vi "SputterTcpSample.vi"() -> ()   [LabVIEW 2021]
doc: "スパッタ制御PC用TCP通信サンプル"
uses:
  SubVI/HallMeasurementStatus.ctl
  SubVI/TcpCommunicationClientCMD.ctl
panel:
  in  "S2_Start":bool
  in  "S2_DataFilePath":path=path "S2_DataFile"
  out "S2_SettingFilePath":path
  out "S2_SampleName":string
  in  "S2_Status":T1
  out "TcpOK?":bool
  in  "S1_Start":bool
  in  "S1_DataFilePath":path=path "S1_DataFile"
  out "S1_SettingFilePath":path
  out "S1_SampleName":string
  in  "S1_Status":T1
  out "ReadData":string
  in  "Send Data":string
  in  "Send":bool
  in  "ポート":u16=8501
  in  "中央PCアドレス":string="localhost"
  in  "停止":bool
  # "スパッタ制御PC用TCP通信サンプル"
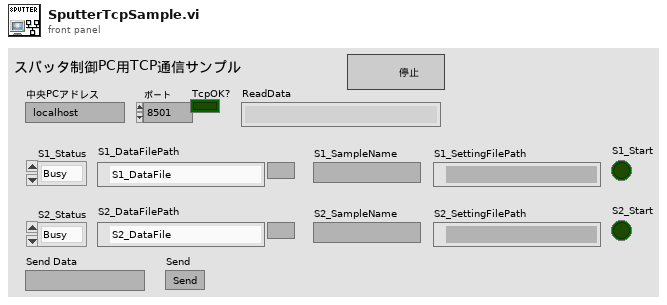
[diagram p1: front panel]
types:
  T1 = typedef "HallMeasurementStatus.ctl" = enum16{"Busy", "Ready", "Done", "Error"}
  T2 = typedef "TcpCommunicationClientCMD.ctl" = enum16{"Read", "Write", "Close"}
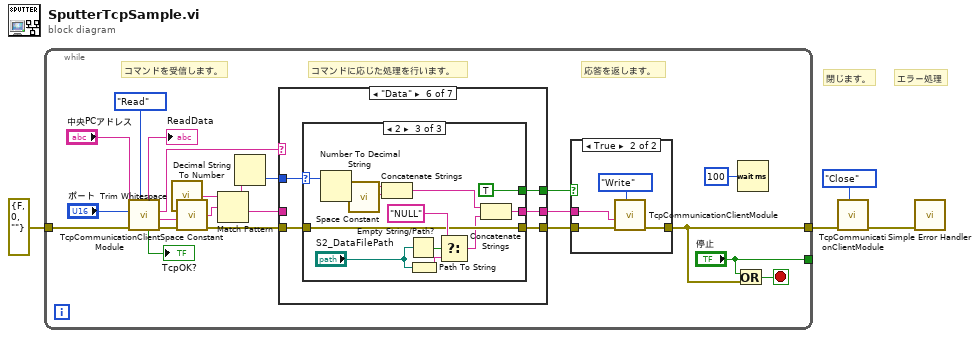
[diagram p0: block diagram]
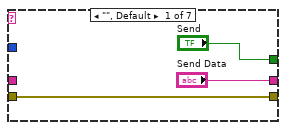
[diagram p3: hidden frame]
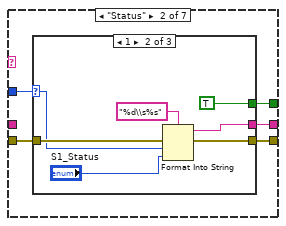
[diagram p4: hidden frame]
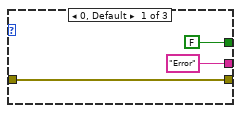
[diagram p5: hidden frame]
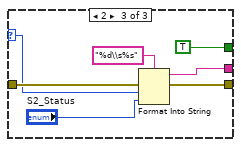
[diagram p6: hidden frame]
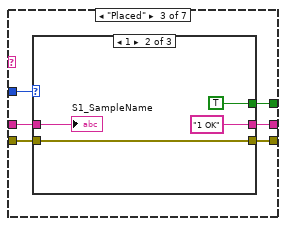
[diagram p7: hidden frame]
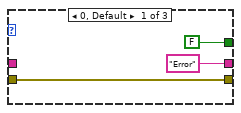
[diagram p8: hidden frame]
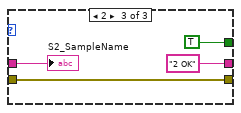
[diagram p9: hidden frame]
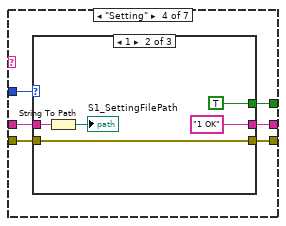
[diagram p10: hidden frame]
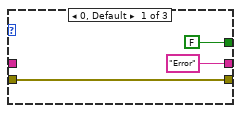
[diagram p11: hidden frame]
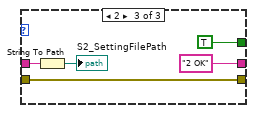
[diagram p12: hidden frame]
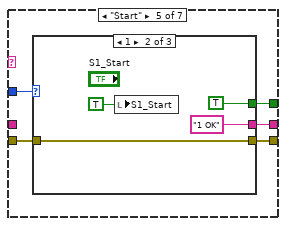
[diagram p13: hidden frame]
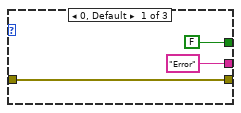
[diagram p14: hidden frame]
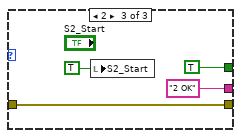
[diagram p15: hidden frame]
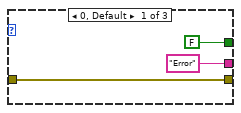
[diagram p16: hidden frame]
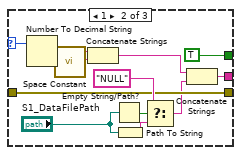
[diagram p17: hidden frame]
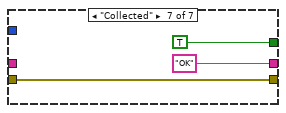
[diagram p18: hidden frame]
diagram:
  # "エラー処理"
  # "閉じます。"
  n1 = while {
    tunnel: ["停止"] -> _
    tunnel: [w14] -> w2
    tunnel: errorcluster {"status"=FALSE, "code"=0, "source"=""} ("エラー入力（エラーなし）") -> [w21]
    stop <- w25 stop-if-true
    # "応答を返します。"
    # "コマンドに応じた処理を行います。"
    # "コマンドを受信します。"
    n2 = call "TcpCommunicationClientModule.vi"("TcpCommunicationClientCMD"=TcpCommunicationClientCMD."Read", "エラー入力（エラーなし）"=w21, "ポート"="ポート", "アドレス"="中央PCアドレス") -> ("エラー出力"=w23:errorcluster, "Data"=w7:string, "Command"=w12:string, "TcpOK?"=→"TcpOK?":bool, "ReadData"=→"ReadData":string)  [unwired: 3 in]
    n3 = call <vilib>:"Trim Whitespace.vi"("string"=w7) -> ("trimmed string"=w8:string)  [unwired: 1 in]
    n4 = call <vilib>:"Space Constant.vi"() -> ("String"=w9:string)
    n5 = Match Pattern(string=w8, regular expression=w9) -> (before substring=w10:string, after substring=w6:string)  [unwired: 1 in, 2 out]
    n6 = Decimal String To Number(string=w10) -> (number=w5:i32)  [unwired: 2 in, 1 out]
    n7 = case shown="\"Data\"" w12 {
      tunnel: w6 -> [_ _ w59 w76 _ _ _]
      tunnel: ["Send Data" w38 w60 w77 w95 w111 "OK" ("Send Data")] -> w16
      tunnel: ["Send" w35 w61 w78 w96 w112 TRUE ("Send")] -> w17
      tunnel: w23 -> [w31 w37 w56 w73 w92 w109 w141]
      tunnel: [w31 w36 w57 w74 w93 w110 w141] -> w15
      tunnel: w5 -> [_ w34 w58 w75 w94 w108 _]
      frame "", Default {
      }
      frame "Status" {
        n8 = case shown="1" w34 {
          selector: w34 -> [_ w42 w50]
          tunnel: ["Error" w47 w55] -> w38
          tunnel: w37 -> [w41 w45 w53]
          tunnel: [w41 w44 w52] -> w36
          tunnel: [FALSE ("Send") TRUE ("Send") TRUE ("Send")] -> w35
          frame 0, Default {
          }
          frame 1 {
            n9 = Format Into String(format string="%d\\s%s" ("形式文字列"), error in=w45, w42, "S1_Status") -> (resulting string=w47:string, error out=w44:errorcluster)  [unwired: 1 in]
          }
          frame 2 {
            n10 = Format Into String(format string="%d\\s%s" ("形式文字列"), error in=w53, w50, "S2_Status") -> (resulting string=w55:string, error out=w52:errorcluster)  [unwired: 1 in]
          }
        }
      }
      frame "Placed" {
        n11 = case shown="1" w58 {
          tunnel: [FALSE ("Send") TRUE ("Send") TRUE ("Send")] -> w61
          tunnel: ["Error" ("Send Data") "1 OK" ("Send Data") "2 OK" ("Send Data")] -> w60
          tunnel: w59 -> [_ w66 w69]
          tunnel: [w64 w65 w70] -> w57
          tunnel: w56 -> [w64 w65 w70]
          frame 0, Default {
          }
          frame 1 {
            "S1_SampleName" <- w66
          }
          frame 2 {
            "S2_SampleName" <- w69
          }
        }
      }
      frame "Setting" {
        n12 = case shown="1" w75 {
          tunnel: [FALSE ("Send") TRUE ("Send") TRUE ("Send")] -> w78
          tunnel: ["Error" ("Send Data") "1 OK" ("Send Data") "2 OK" ("Send Data")] -> w77
          tunnel: w76 -> [_ w84 w89]
          tunnel: [w81 w82 w88] -> w74
          tunnel: w73 -> [w81 w82 w88]
          frame 0, Default {
          }
          frame 1 {
            n13 = String To Path(string=w84) -> (path=→"S1_SettingFilePath":path)
          }
          frame 2 {
            n14 = String To Path(string=w89) -> (path=→"S2_SettingFilePath":path)
          }
        }
      }
      frame "Start" {
        n15 = case shown="1" w94 {
          tunnel: [FALSE ("Send") TRUE ("Send") TRUE ("Send")] -> w96
          tunnel: ["Error" ("Send Data") "1 OK" ("Send Data") "2 OK" ("Send Data")] -> w95
          tunnel: [w99 w100 w104] -> w93
          tunnel: w92 -> [w99 w100 w104]
          frame 0, Default {
          }
          frame 1 {
            n16 = local write "S1_Start"(TRUE) -> ()
          }
          frame 2 {
            n17 = local write "S2_Start"(TRUE) -> ()
          }
        }
      }
      frame "Data" {
        n18 = case shown="2" w108 {
          selector: w108 -> [_ w118 w130]
          tunnel: [FALSE ("Send") TRUE ("Send") TRUE ("Send")] -> w112
          tunnel: ["Error" ("t") w116 w128] -> w111
          tunnel: [w115 w122 w135] -> w110
          tunnel: w109 -> [w115 w122 w135]
          frame 0, Default {
          }
          frame 1 {
            n19 = Number To Decimal String(number=w118) -> (decimal integer string=w119:string)  [unwired: 1 in]
            n20 = call <vilib>:"Space Constant.vi"() -> ("String"=w120:string)
            n21 = Concatenate Strings(w119, w120) -> (w121:string)
            n22 = Empty String/Path?(string/path="S1_DataFilePath") -> (empty?=w125:bool)
            n23 = Path To String(path="S1_DataFilePath") -> (string=w124:string)
            n24 = Select(t="NULL", s=w125, f=w124) -> (s? t:f=w117:string)
            n25 = Concatenate Strings(w121, w117) -> (w116:string)
          }
          frame 2 {
            n26 = Number To Decimal String(number=w130) -> (decimal integer string=w131:string)  [unwired: 1 in]
            n27 = call <vilib>:"Space Constant.vi"() -> ("String"=w132:string)
            n28 = Concatenate Strings(w131, w132) -> (w133:string)
            n29 = Empty String/Path?(string/path="S2_DataFilePath") -> (empty?=w138:bool)
            n30 = Path To String(path="S2_DataFilePath") -> (string=w137:string)
            n31 = Select(t="NULL", s=w138, f=w137) -> (s? t:f=w129:string)
            n32 = Concatenate Strings(w133, w129) -> (w128:string)
          }
        }
      }
      frame "Collected" {
      }
    }
    n33 = case shown="True" w17 {
      tunnel: w15 -> [w26 w30]
      tunnel: [w26 w29] -> w14
      tunnel: w16 -> [_ w27]
      frame False {
      }
      frame True {
        n34 = call "TcpCommunicationClientModule.vi"("TcpCommunicationClientCMD"=TcpCommunicationClientCMD."Write", "エラー入力（エラーなし）"=w30, "WriteData"=w27) -> ("エラー出力"=w29:errorcluster)  [unwired: 4 in, 4 out]
      }
    }
    n35 = Or(x="停止", y=w14) -> (x .or. y?=w25:bool)
    n36 = Wait (ms)(milliseconds to wait=u32 100 ("ミリ秒待機時間")) -> ()  [unwired: 1 out]
  }
  n37 = call "TcpCommunicationClientModule.vi"("TcpCommunicationClientCMD"=TcpCommunicationClientCMD."Close", "エラー入力（エラーなし）"=w2) -> ("エラー出力"=w1:errorcluster)  [unwired: 5 in, 4 out]
  n38 = call <vilib>:"Simple Error Handler.vi"("error in (no error)"=w1) -> ()  [unwired: 1 in, 8 out]
